vi "VIP_Post-Uninstall Custom Action.vi"(10 "Variant":variant) -> (0 "error out":errorcluster)   [LabVIEW 2020]
uses:
  <vilib>/zip/NI_Unzip.lvlib
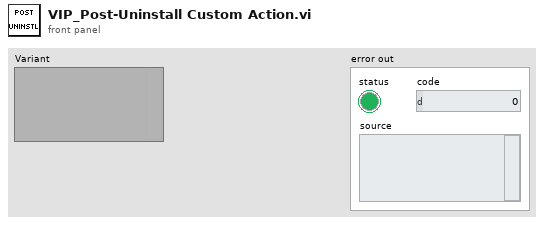
[diagram p1: front panel]
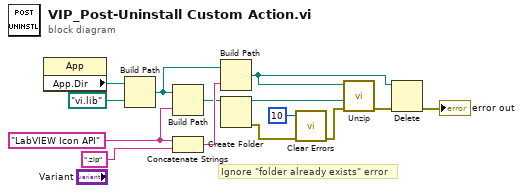
[diagram p0: block diagram]
diagram:
  w7 = "LabVIEW Icon API"
  # "Ignore \"folder already exists\" error"
  n1 = property class="App"() -> ("App.Dir"=w1:path)  [unwired: 2 in, 2 out]
  n2 = Build Path(base path=w1, name or relative path=path "vi.lib" ("symbolic path")) -> (appended path=w5:path)
  n3 = Build Path(base path=w5, name or relative path=w7) -> (appended path=w2:path)
  n4 = Concatenate Strings(w7, ".zip" ("string")) -> (w4:string)
  n5 = Build Path(base path=w5, name or relative path=w4) -> (appended path=w3:path)
  n6 = Create Folder(path (use dialog)=w2) -> (created path=w10:path, error out=w14:errorcluster)  [unwired: 2 in, 1 out]
  n7 = call <vilib>:"Clear Errors.vi"("error in (no error)"=w14, "specific error code to clear (0: all)"=10) -> ("error out"=w13:errorcluster)  [unwired: 4 in, 1 out]
  n8 = call <vilib>:"Unzip.vi"("error in (no error)"=w13, "Target directory (same as Zip file if empty)"=w10, "Zip file"=w3) -> ("error out"=w12:errorcluster)  [unwired: 6 in, 2 out]
  n9 = Delete(path (use dialog)=w3, error in=w12) -> (error out=→"error out":errorcluster)  [unwired: 3 in, 2 out]
